vi "EnFlo_Tunnel_Global.vi"() -> ()   [LabVIEW 2017]
panel:
  in  "Minimum Shaft RPM":dbl=45.0
  in  "Minimum Ref Velocity":dbl=0.1
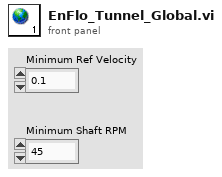
[diagram p1: front panel]
diagram:
